vi "TCH Golbal.vi"() -> ()   [LabVIEW 2017]
panel:
  in  "秒进位":dbl
  in  "SweepCounter":i32
  in  "MouseFlag":bool
  in  "GetDataQE":bool
  in  "CloseSetVI":bool
  out "图像数据":i32[][](array[numeric])
  in  "read time":dbl
  in  "是否获取图片":dbl
  in  "Getimage flg":bool
  in  "曝光时间":dbl
  in  "Resolution flg":bool
  in  "位置保存次数":i32
  in  "结果保存次数":i32
  in  "累积位置":cluster{"X":i32, "Y":i32, "Z":i32}
  in  "ZeroFlag":cluster{"X":bool, "Y":bool, "Z":bool}
  in  "位置记录":cluster{"X":i32, "Y":i32, "Z":i32}[](array[cluster])
  in  "Clear位置":cluster{"X":i32, "Y":i32, "Z":i32}
  in  "原点":cluster{"X":i32, "Y":i32, "z":i32}
  in  "ExposureFlag":bool
  in  "Manual Color Palette":cluster{"Red":u8, "Green":u8, "Blue":u8}[](array[cluster])=[{"Red"=0, "Green"=0, "Blue"=0}, {"Red"=0, "Green"=0, "Blue"=0}, {"Red"=0, "Green"=0, "Blue"=0}, {"Red"=0, "Green"=0, "Blue"=0}, {"Red"=0, "Green"=0, "Blue"=0}, {"Red"=0, "Green"=0, "Blue"=0}, {"Red"=0, "Green"=0, "Blue"=0}, {"Red"=0, "Green"=0, "Blue"=0}, {"Red"=0, "Green"=0, "Blue"=0}, {"Red"=0, "Green"=0, "Blue"=0}, {"Red"=0, "Green"=0, "Blue"=0}, {"Red"=0, "Green"=0, "Blue"=0}, {"Red"=0, "Green"=0, "Blue"=0}, {"Red"=0, "Green"=0, "Blue"=0}, {"Red"=0, "Green"=0, "Blue"=0}, {"Red"=0, "Green"=0, "Blue"=0}, {"Red"=0, "Green"=0, "Blue"=0}, {"Red"=0, "Green"=0, "Blue"=0}, {"Red"=0, "Green"=0, "Blue"=0}, {"Red"=0, "Green"=0, "Blue"=0}, {"Red"=0, "Green"=0, "Blue"=0}, {"Red"=0, "Green"=0, "Blue"=0}, {"Red"=0, "Green"=0, "Blue"=0}, {"Red"=0, "Green"=0, "Blue"=0}, {"Red"=0, "Green"=0, "Blue"=0}, {"Red"=0, "Green"=0, "Blue"=0}, {"Red"=0, "Green"=0, "Blue"=0}, {"Red"=0, "Green"=0, "Blue"=0}, {"Red"=0, "Green"=0, "Blue"=0}, {"Red"=0, "Green"=0, "Blue"=0}, {"Red"=0, "Green"=0, "Blue"=0}, {"Red"=0, "Green"=0, "Blue"=0}, {"Red"=0, "Green"=0, "Blue"=0}, {"Red"=0, "Green"=0, "Blue"=0}, {"Red"=0, "Green"=0, "Blue"=0}, {"Red"=0, "Green"=0, "Blue"=0}, {"Red"=0, "Green"=0, "Blue"=0}, {"Red"=0, "Green"=0, "Blue"=0}, {"Red"=0, "Green"=0, "Blue"=0}, {"Red"=0, "Green"=0, "Blue"=0}, {"Red"=0, "Green"=0, "Blue"=0}, {"Red"=0, "Green"=0, "Blue"=0}, {"Red"=0, "Green"=0, "Blue"=0}, {"Red"=0, "Green"=0, "Blue"=0}, {"Red"=0, "Green"=0, "Blue"=0}, {"Red"=0, "Green"=0, "Blue"=0}, {"Red"=0, "Green"=0, "Blue"=0}, {"Red"=0, "Green"=0, "Blue"=0}, {"Red"=0, "Green"=0, "Blue"=0}, {"Red"=0, "Green"=0, "Blue"=0}, {"Red"=0, "Green"=0, "Blue"=0}, {"Red"=0, "Green"=0, "Blue"=0}, {"Red"=0, "Green"=0, "Blue"=0}, {"Red"=0, "Green"=0, "Blue"=0}, {"Red"=0, "Green"=0, "Blue"=0}, {"Red"=0, "Green"=0, "Blue"=0}, {"Red"=0, "Green"=0, "Blue"=0}, {"Red"=0, "Green"=0, "Blue"=0}, {"Red"=0, "Green"=0, "Blue"=0}, {"Red"=0, "Green"=0, "Blue"=0}, {"Red"=0, "Green"=0, "Blue"=0}, {"Red"=0, "Green"=0, "Blue"=0}, {"Red"=0, "Green"=0, "Blue"=0}, {"Red"=0, "Green"=0, "Blue"=0}, {"Red"=0, "Green"=0, "Blue"=0}, {"Red"=0, "Green"=0, "Blue"=0}, {"Red"=0, "Green"=0, "Blue"=0}, {"Red"=0, "Green"=0, "Blue"=0}, {"Red"=0, "Green"=0, "Blue"=0}, {"Red"=0, "Green"=0, "Blue"=0}, {"Red"=0, "Green"=0, "Blue"=0}, {"Red"=0, "Green"=0, "Blue"=0}, {"Red"=0, "Green"=0, "Blue"=0}, {"Red"=0, "Green"=0, "Blue"=0}, {"Red"=0, "Green"=0, "Blue"=0}, {"Red"=0, "Green"=0, "Blue"=0}, {"Red"=0, "Green"=0, "Blue"=0}, {"Red"=0, "Green"=0, "Blue"=0}, {"Red"=0, "Green"=0, "Blue"=0}, {"Red"=0, "Green"=0, "Blue"=0}, {"Red"=0, "Green"=0, "Blue"=0}, {"Red"=0, "Green"=0, "Blue"=0}, {"Red"=0, "Green"=0, "Blue"=0}, {"Red"=0, "Green"=0, "Blue"=0}, {"Red"=0, "Green"=0, "Blue"=0}, {"Red"=0, "Green"=0, "Blue"=0}, {"Red"=0, "Green"=0, "Blue"=0}, {"Red"=0, "Green"=0, "Blue"=0}, {"Red"=0, "Green"=0, "Blue"=0}, {"Red"=0, "Green"=0, "Blue"=0}, {"Red"=0, "Green"=0, "Blue"=0}, {"Red"=0, "Green"=0, "Blue"=0}, {"Red"=0, "Green"=0, "Blue"=0}, {"Red"=0, "Green"=0, "Blue"=0}, {"Red"=0, "Green"=0, "Blue"=0}, {"Red"=0, "Green"=0, "Blue"=0}, {"Red"=0, "Green"=0, "Blue"=0}, {"Red"=0, "Green"=0, "Blue"=0}, {"Red"=0, "Green"=0, "Blue"=0}, {"Red"=0, "Green"=0, "Blue"=0}, {"Red"=0, "Green"=0, "Blue"=0}, {"Red"=0, "Green"=0, "Blue"=0}, {"Red"=0, "Green"=0, "Blue"=0}, {"Red"=0, "Green"=0, "Blue"=0}, {"Red"=0, "Green"=0, "Blue"=0}, {"Red"=0, "Green"=0, "Blue"=0}, {"Red"=0, "Green"=0, "Blue"=0}, {"Red"=0, "Green"=0, "Blue"=0}, {"Red"=0, "Green"=0, "Blue"=0}, {"Red"=0, "Green"=0, "Blue"=0}, {"Red"=0, "Green"=0, "Blue"=0}, {"Red"=0, "Green"=0, "Blue"=0}, {"Red"=0, "Green"=0, "Blue"=0}, {"Red"=0, "Green"=0, "Blue"=0}, {"Red"=0, "Green"=0, "Blue"=0}, {"Red"=0, "Green"=0, "Blue"=0}, {"Red"=0, "Green"=0, "Blue"=0}, {"Red"=0, "Green"=0, "Blue"=0}, {"Red"=0, "Green"=0, "Blue"=0}, {"Red"=0, "Green"=0, "Blue"=0}, {"Red"=0, "Green"=0, "Blue"=0}, {"Red"=0, "Green"=0, "Blue"=0}, {"Red"=0, "Green"=0, "Blue"=0}, {"Red"=0, "Green"=0, "Blue"=0}, {"Red"=0, "Green"=0, "Blue"=0}, {"Red"=0, "Green"=0, "Blue"=0}, {"Red"=0, "Green"=0, "Blue"=0}, {"Red"=0, "Green"=0, "Blue"=0}, {"Red"=0, "Green"=255, "Blue"=0}, {"Red"=4, "Green"=255, "Blue"=0}, {"Red"=8, "Green"=255, "Blue"=0}, {"Red"=12, "Green"=255, "Blue"=0}, {"Red"=16, "Green"=255, "Blue"=0}, {"Red"=20, "Green"=255, "Blue"=0}, {"Red"=24, "Green"=255, "Blue"=0}, {"Red"=28, "Green"=255, "Blue"=0}, {"Red"=32, "Green"=255, "Blue"=0}, {"Red"=36, "Green"=255, "Blue"=0}, {"Red"=40, "Green"=255, "Blue"=0}, {"Red"=44, "Green"=255, "Blue"=0}, {"Red"=48, "Green"=255, "Blue"=0}, {"Red"=52, "Green"=255, "Blue"=0}, {"Red"=56, "Green"=255, "Blue"=0}, {"Red"=60, "Green"=255, "Blue"=0}, {"Red"=64, "Green"=255, "Blue"=0}, {"Red"=68, "Green"=255, "Blue"=0}, {"Red"=72, "Green"=255, "Blue"=0}, {"Red"=76, "Green"=255, "Blue"=0}, {"Red"=80, "Green"=255, "Blue"=0}, {"Red"=84, "Green"=255, "Blue"=0}, {"Red"=88, "Green"=255, "Blue"=0}, {"Red"=92, "Green"=255, "Blue"=0}, {"Red"=96, "Green"=255, "Blue"=0}, {"Red"=100, "Green"=255, "Blue"=0}, {"Red"=104, "Green"=255, "Blue"=0}, {"Red"=108, "Green"=255, "Blue"=0}, {"Red"=112, "Green"=255, "Blue"=0}, {"Red"=116, "Green"=255, "Blue"=0}, {"Red"=120, "Green"=255, "Blue"=0}, {"Red"=124, "Green"=255, "Blue"=0}, {"Red"=128, "Green"=255, "Blue"=0}, {"Red"=132, "Green"=255, "Blue"=0}, {"Red"=136, "Green"=255, "Blue"=0}, {"Red"=140, "Green"=255, "Blue"=0}, {"Red"=144, "Green"=255, "Blue"=0}, {"Red"=148, "Green"=255, "Blue"=0}, {"Red"=152, "Green"=255, "Blue"=0}, {"Red"=156, "Green"=255, "Blue"=0}, {"Red"=160, "Green"=255, "Blue"=0}, {"Red"=164, "Green"=255, "Blue"=0}, {"Red"=168, "Green"=255, "Blue"=0}, {"Red"=172, "Green"=255, "Blue"=0}, {"Red"=176, "Green"=255, "Blue"=0}, {"Red"=180, "Green"=255, "Blue"=0}, {"Red"=184, "Green"=255, "Blue"=0}, {"Red"=188, "Green"=255, "Blue"=0}, {"Red"=192, "Green"=255, "Blue"=0}, {"Red"=196, "Green"=255, "Blue"=0}, {"Red"=200, "Green"=255, "Blue"=0}, {"Red"=204, "Green"=255, "Blue"=0}, {"Red"=208, "Green"=255, "Blue"=0}, {"Red"=212, "Green"=255, "Blue"=0}, {"Red"=216, "Green"=255, "Blue"=0}, {"Red"=220, "Green"=255, "Blue"=0}, {"Red"=224, "Green"=255, "Blue"=0}, {"Red"=228, "Green"=255, "Blue"=0}, {"Red"=232, "Green"=255, "Blue"=0}, {"Red"=236, "Green"=255, "Blue"=0}, {"Red"=240, "Green"=255, "Blue"=0}, {"Red"=244, "Green"=255, "Blue"=0}, {"Red"=248, "Green"=255, "Blue"=0}, {"Red"=252, "Green"=255, "Blue"=0}, {"Red"=255, "Green"=255, "Blue"=0}, {"Red"=255, "Green"=251, "Blue"=0}, {"Red"=255, "Green"=247, "Blue"=0}, {"Red"=255, "Green"=243, "Blue"=0}, {"Red"=255, "Green"=239, "Blue"=0}, {"Red"=255, "Green"=235, "Blue"=0}, {"Red"=255, "Green"=231, "Blue"=0}, {"Red"=255, "Green"=227, "Blue"=0}, {"Red"=255, "Green"=223, "Blue"=0}, {"Red"=255, "Green"=219, "Blue"=0}, {"Red"=255, "Green"=215, "Blue"=0}, {"Red"=255, "Green"=211, "Blue"=0}, {"Red"=255, "Green"=207, "Blue"=0}, {"Red"=255, "Green"=203, "Blue"=0}, {"Red"=255, "Green"=199, "Blue"=0}, {"Red"=255, "Green"=195, "Blue"=0}, {"Red"=255, "Green"=191, "Blue"=0}, {"Red"=255, "Green"=187, "Blue"=0}, {"Red"=255, "Green"=183, "Blue"=0}, {"Red"=255, "Green"=179, "Blue"=0}, {"Red"=255, "Green"=175, "Blue"=0}, {"Red"=255, "Green"=171, "Blue"=0}, {"Red"=255, "Green"=167, "Blue"=0}, {"Red"=255, "Green"=163, "Blue"=0}, {"Red"=255, "Green"=159, "Blue"=0}, {"Red"=255, "Green"=155, "Blue"=0}, {"Red"=255, "Green"=151, "Blue"=0}, {"Red"=255, "Green"=147, "Blue"=0}, {"Red"=255, "Green"=143, "Blue"=0}, {"Red"=255, "Green"=139, "Blue"=0}, {"Red"=255, "Green"=135, "Blue"=0}, {"Red"=255, "Green"=131, "Blue"=0}, {"Red"=255, "Green"=127, "Blue"=0}, {"Red"=255, "Green"=123, "Blue"=0}, {"Red"=255, "Green"=119, "Blue"=0}, {"Red"=255, "Green"=115, "Blue"=0}, {"Red"=255, "Green"=111, "Blue"=0}, {"Red"=255, "Green"=107, "Blue"=0}, {"Red"=255, "Green"=103, "Blue"=0}, {"Red"=255, "Green"=99, "Blue"=0}, {"Red"=255, "Green"=95, "Blue"=0}, {"Red"=255, "Green"=91, "Blue"=0}, {"Red"=255, "Green"=87, "Blue"=0}, {"Red"=255, "Green"=83, "Blue"=0}, {"Red"=255, "Green"=79, "Blue"=0}, {"Red"=255, "Green"=75, "Blue"=0}, {"Red"=255, "Green"=71, "Blue"=0}, {"Red"=255, "Green"=67, "Blue"=0}, {"Red"=255, "Green"=63, "Blue"=0}, {"Red"=255, "Green"=59, "Blue"=0}, {"Red"=255, "Green"=55, "Blue"=0}, {"Red"=255, "Green"=51, "Blue"=0}, {"Red"=255, "Green"=47, "Blue"=0}, {"Red"=255, "Green"=43, "Blue"=0}, {"Red"=255, "Green"=39, "Blue"=0}, {"Red"=255, "Green"=35, "Blue"=0}, {"Red"=255, "Green"=31, "Blue"=0}, {"Red"=255, "Green"=27, "Blue"=0}, {"Red"=255, "Green"=23, "Blue"=0}, {"Red"=255, "Green"=19, "Blue"=0}, {"Red"=255, "Green"=15, "Blue"=0}, {"Red"=255, "Green"=11, "Blue"=0}, {"Red"=255, "Green"=7, "Blue"=0}, {"Red"=255, "Green"=3, "Blue"=0}]
  in  "Auto Color Palette":cluster{"Red":u8, "Green":u8, "Blue":u8}[](array[cluster])=[{"Red"=0, "Green"=0, "Blue"=0}, {"Red"=0, "Green"=0, "Blue"=0}, {"Red"=0, "Green"=0, "Blue"=0}, {"Red"=0, "Green"=0, "Blue"=0}, {"Red"=0, "Green"=0, "Blue"=0}, {"Red"=0, "Green"=0, "Blue"=0}, {"Red"=0, "Green"=0, "Blue"=0}, {"Red"=0, "Green"=0, "Blue"=0}, {"Red"=0, "Green"=0, "Blue"=0}, {"Red"=0, "Green"=0, "Blue"=0}, {"Red"=0, "Green"=0, "Blue"=0}, {"Red"=0, "Green"=0, "Blue"=0}, {"Red"=0, "Green"=0, "Blue"=0}, {"Red"=0, "Green"=0, "Blue"=0}, {"Red"=0, "Green"=0, "Blue"=0}, {"Red"=0, "Green"=0, "Blue"=0}, {"Red"=0, "Green"=0, "Blue"=0}, {"Red"=0, "Green"=0, "Blue"=0}, {"Red"=0, "Green"=0, "Blue"=0}, {"Red"=0, "Green"=0, "Blue"=0}, {"Red"=0, "Green"=0, "Blue"=0}, {"Red"=0, "Green"=0, "Blue"=0}, {"Red"=0, "Green"=0, "Blue"=0}, {"Red"=0, "Green"=0, "Blue"=0}, {"Red"=0, "Green"=0, "Blue"=0}, {"Red"=0, "Green"=0, "Blue"=0}, {"Red"=0, "Green"=0, "Blue"=0}, {"Red"=0, "Green"=0, "Blue"=0}, {"Red"=0, "Green"=0, "Blue"=0}, {"Red"=0, "Green"=0, "Blue"=0}, {"Red"=0, "Green"=0, "Blue"=0}, {"Red"=0, "Green"=0, "Blue"=0}, {"Red"=0, "Green"=0, "Blue"=0}, {"Red"=0, "Green"=0, "Blue"=0}, {"Red"=0, "Green"=0, "Blue"=0}, {"Red"=0, "Green"=0, "Blue"=0}, {"Red"=0, "Green"=0, "Blue"=0}, {"Red"=0, "Green"=0, "Blue"=0}, {"Red"=0, "Green"=0, "Blue"=0}, {"Red"=0, "Green"=0, "Blue"=0}, {"Red"=0, "Green"=0, "Blue"=0}, {"Red"=0, "Green"=0, "Blue"=0}, {"Red"=0, "Green"=0, "Blue"=0}, {"Red"=0, "Green"=0, "Blue"=0}, {"Red"=0, "Green"=0, "Blue"=0}, {"Red"=0, "Green"=0, "Blue"=0}, {"Red"=0, "Green"=0, "Blue"=0}, {"Red"=0, "Green"=0, "Blue"=0}, {"Red"=0, "Green"=0, "Blue"=0}, {"Red"=0, "Green"=0, "Blue"=0}, {"Red"=0, "Green"=0, "Blue"=0}, {"Red"=0, "Green"=0, "Blue"=0}, {"Red"=0, "Green"=0, "Blue"=0}, {"Red"=0, "Green"=0, "Blue"=0}, {"Red"=0, "Green"=0, "Blue"=0}, {"Red"=0, "Green"=0, "Blue"=0}, {"Red"=0, "Green"=0, "Blue"=0}, {"Red"=0, "Green"=0, "Blue"=0}, {"Red"=0, "Green"=0, "Blue"=0}, {"Red"=0, "Green"=0, "Blue"=0}, {"Red"=0, "Green"=0, "Blue"=0}, {"Red"=0, "Green"=0, "Blue"=0}, {"Red"=0, "Green"=0, "Blue"=0}, {"Red"=0, "Green"=0, "Blue"=0}, {"Red"=0, "Green"=0, "Blue"=0}, {"Red"=0, "Green"=0, "Blue"=0}, {"Red"=0, "Green"=0, "Blue"=0}, {"Red"=0, "Green"=0, "Blue"=0}, {"Red"=0, "Green"=0, "Blue"=0}, {"Red"=0, "Green"=0, "Blue"=0}, {"Red"=0, "Green"=0, "Blue"=0}, {"Red"=0, "Green"=0, "Blue"=0}, {"Red"=0, "Green"=0, "Blue"=0}, {"Red"=0, "Green"=0, "Blue"=0}, {"Red"=0, "Green"=0, "Blue"=0}, {"Red"=0, "Green"=0, "Blue"=0}, {"Red"=0, "Green"=0, "Blue"=0}, {"Red"=0, "Green"=0, "Blue"=0}, {"Red"=0, "Green"=0, "Blue"=0}, {"Red"=0, "Green"=0, "Blue"=0}, {"Red"=0, "Green"=0, "Blue"=0}, {"Red"=0, "Green"=0, "Blue"=0}, {"Red"=0, "Green"=0, "Blue"=0}, {"Red"=0, "Green"=0, "Blue"=0}, {"Red"=0, "Green"=0, "Blue"=0}, {"Red"=0, "Green"=0, "Blue"=0}, {"Red"=0, "Green"=0, "Blue"=0}, {"Red"=0, "Green"=0, "Blue"=0}, {"Red"=0, "Green"=0, "Blue"=0}, {"Red"=0, "Green"=0, "Blue"=0}, {"Red"=0, "Green"=0, "Blue"=0}, {"Red"=0, "Green"=0, "Blue"=0}, {"Red"=0, "Green"=0, "Blue"=0}, {"Red"=0, "Green"=0, "Blue"=0}, {"Red"=0, "Green"=0, "Blue"=0}, {"Red"=0, "Green"=0, "Blue"=0}, {"Red"=0, "Green"=0, "Blue"=0}, {"Red"=0, "Green"=0, "Blue"=0}, {"Red"=0, "Green"=0, "Blue"=0}, {"Red"=0, "Green"=0, "Blue"=0}, {"Red"=0, "Green"=0, "Blue"=0}, {"Red"=0, "Green"=0, "Blue"=0}, {"Red"=0, "Green"=0, "Blue"=0}, {"Red"=0, "Green"=0, "Blue"=0}, {"Red"=0, "Green"=0, "Blue"=0}, {"Red"=0, "Green"=0, "Blue"=0}, {"Red"=0, "Green"=0, "Blue"=0}, {"Red"=0, "Green"=0, "Blue"=0}, {"Red"=0, "Green"=0, "Blue"=0}, {"Red"=0, "Green"=0, "Blue"=0}, {"Red"=0, "Green"=0, "Blue"=0}, {"Red"=0, "Green"=0, "Blue"=0}, {"Red"=0, "Green"=0, "Blue"=0}, {"Red"=0, "Green"=0, "Blue"=0}, {"Red"=0, "Green"=0, "Blue"=0}, {"Red"=0, "Green"=0, "Blue"=0}, {"Red"=0, "Green"=0, "Blue"=0}, {"Red"=0, "Green"=0, "Blue"=0}, {"Red"=0, "Green"=0, "Blue"=0}, {"Red"=0, "Green"=0, "Blue"=0}, {"Red"=0, "Green"=0, "Blue"=0}, {"Red"=0, "Green"=0, "Blue"=0}, {"Red"=0, "Green"=0, "Blue"=0}, {"Red"=0, "Green"=0, "Blue"=0}, {"Red"=0, "Green"=0, "Blue"=0}, {"Red"=0, "Green"=0, "Blue"=0}, {"Red"=0, "Green"=0, "Blue"=0}, {"Red"=0, "Green"=0, "Blue"=0}, {"Red"=0, "Green"=255, "Blue"=0}, {"Red"=4, "Green"=255, "Blue"=0}, {"Red"=8, "Green"=255, "Blue"=0}, {"Red"=12, "Green"=255, "Blue"=0}, {"Red"=16, "Green"=255, "Blue"=0}, {"Red"=20, "Green"=255, "Blue"=0}, {"Red"=24, "Green"=255, "Blue"=0}, {"Red"=28, "Green"=255, "Blue"=0}, {"Red"=32, "Green"=255, "Blue"=0}, {"Red"=36, "Green"=255, "Blue"=0}, {"Red"=40, "Green"=255, "Blue"=0}, {"Red"=44, "Green"=255, "Blue"=0}, {"Red"=48, "Green"=255, "Blue"=0}, {"Red"=52, "Green"=255, "Blue"=0}, {"Red"=56, "Green"=255, "Blue"=0}, {"Red"=60, "Green"=255, "Blue"=0}, {"Red"=64, "Green"=255, "Blue"=0}, {"Red"=68, "Green"=255, "Blue"=0}, {"Red"=72, "Green"=255, "Blue"=0}, {"Red"=76, "Green"=255, "Blue"=0}, {"Red"=80, "Green"=255, "Blue"=0}, {"Red"=84, "Green"=255, "Blue"=0}, {"Red"=88, "Green"=255, "Blue"=0}, {"Red"=92, "Green"=255, "Blue"=0}, {"Red"=96, "Green"=255, "Blue"=0}, {"Red"=100, "Green"=255, "Blue"=0}, {"Red"=104, "Green"=255, "Blue"=0}, {"Red"=108, "Green"=255, "Blue"=0}, {"Red"=112, "Green"=255, "Blue"=0}, {"Red"=116, "Green"=255, "Blue"=0}, {"Red"=120, "Green"=255, "Blue"=0}, {"Red"=124, "Green"=255, "Blue"=0}, {"Red"=128, "Green"=255, "Blue"=0}, {"Red"=132, "Green"=255, "Blue"=0}, {"Red"=136, "Green"=255, "Blue"=0}, {"Red"=140, "Green"=255, "Blue"=0}, {"Red"=144, "Green"=255, "Blue"=0}, {"Red"=148, "Green"=255, "Blue"=0}, {"Red"=152, "Green"=255, "Blue"=0}, {"Red"=156, "Green"=255, "Blue"=0}, {"Red"=160, "Green"=255, "Blue"=0}, {"Red"=164, "Green"=255, "Blue"=0}, {"Red"=168, "Green"=255, "Blue"=0}, {"Red"=172, "Green"=255, "Blue"=0}, {"Red"=176, "Green"=255, "Blue"=0}, {"Red"=180, "Green"=255, "Blue"=0}, {"Red"=184, "Green"=255, "Blue"=0}, {"Red"=188, "Green"=255, "Blue"=0}, {"Red"=192, "Green"=255, "Blue"=0}, {"Red"=196, "Green"=255, "Blue"=0}, {"Red"=200, "Green"=255, "Blue"=0}, {"Red"=204, "Green"=255, "Blue"=0}, {"Red"=208, "Green"=255, "Blue"=0}, {"Red"=212, "Green"=255, "Blue"=0}, {"Red"=216, "Green"=255, "Blue"=0}, {"Red"=220, "Green"=255, "Blue"=0}, {"Red"=224, "Green"=255, "Blue"=0}, {"Red"=228, "Green"=255, "Blue"=0}, {"Red"=232, "Green"=255, "Blue"=0}, {"Red"=236, "Green"=255, "Blue"=0}, {"Red"=240, "Green"=255, "Blue"=0}, {"Red"=244, "Green"=255, "Blue"=0}, {"Red"=248, "Green"=255, "Blue"=0}, {"Red"=252, "Green"=255, "Blue"=0}, {"Red"=255, "Green"=255, "Blue"=0}, {"Red"=255, "Green"=251, "Blue"=0}, {"Red"=255, "Green"=247, "Blue"=0}, {"Red"=255, "Green"=243, "Blue"=0}, {"Red"=255, "Green"=239, "Blue"=0}, {"Red"=255, "Green"=235, "Blue"=0}, {"Red"=255, "Green"=231, "Blue"=0}, {"Red"=255, "Green"=227, "Blue"=0}, {"Red"=255, "Green"=223, "Blue"=0}, {"Red"=255, "Green"=219, "Blue"=0}, {"Red"=255, "Green"=215, "Blue"=0}, {"Red"=255, "Green"=211, "Blue"=0}, {"Red"=255, "Green"=207, "Blue"=0}, {"Red"=255, "Green"=203, "Blue"=0}, {"Red"=255, "Green"=199, "Blue"=0}, {"Red"=255, "Green"=195, "Blue"=0}, {"Red"=255, "Green"=191, "Blue"=0}, {"Red"=255, "Green"=187, "Blue"=0}, {"Red"=255, "Green"=183, "Blue"=0}, {"Red"=255, "Green"=179, "Blue"=0}, {"Red"=255, "Green"=175, "Blue"=0}, {"Red"=255, "Green"=171, "Blue"=0}, {"Red"=255, "Green"=167, "Blue"=0}, {"Red"=255, "Green"=163, "Blue"=0}, {"Red"=255, "Green"=159, "Blue"=0}, {"Red"=255, "Green"=155, "Blue"=0}, {"Red"=255, "Green"=151, "Blue"=0}, {"Red"=255, "Green"=147, "Blue"=0}, {"Red"=255, "Green"=143, "Blue"=0}, {"Red"=255, "Green"=139, "Blue"=0}, {"Red"=255, "Green"=135, "Blue"=0}, {"Red"=255, "Green"=131, "Blue"=0}, {"Red"=255, "Green"=127, "Blue"=0}, {"Red"=255, "Green"=123, "Blue"=0}, {"Red"=255, "Green"=119, "Blue"=0}, {"Red"=255, "Green"=115, "Blue"=0}, {"Red"=255, "Green"=111, "Blue"=0}, {"Red"=255, "Green"=107, "Blue"=0}, {"Red"=255, "Green"=103, "Blue"=0}, {"Red"=255, "Green"=99, "Blue"=0}, {"Red"=255, "Green"=95, "Blue"=0}, {"Red"=255, "Green"=91, "Blue"=0}, {"Red"=255, "Green"=87, "Blue"=0}, {"Red"=255, "Green"=83, "Blue"=0}, {"Red"=255, "Green"=79, "Blue"=0}, {"Red"=255, "Green"=75, "Blue"=0}, {"Red"=255, "Green"=71, "Blue"=0}, {"Red"=255, "Green"=67, "Blue"=0}, {"Red"=255, "Green"=63, "Blue"=0}, {"Red"=255, "Green"=59, "Blue"=0}, {"Red"=255, "Green"=55, "Blue"=0}, {"Red"=255, "Green"=51, "Blue"=0}, {"Red"=255, "Green"=47, "Blue"=0}, {"Red"=255, "Green"=43, "Blue"=0}, {"Red"=255, "Green"=39, "Blue"=0}, {"Red"=255, "Green"=35, "Blue"=0}, {"Red"=255, "Green"=31, "Blue"=0}, {"Red"=255, "Green"=27, "Blue"=0}, {"Red"=255, "Green"=23, "Blue"=0}, {"Red"=255, "Green"=19, "Blue"=0}, {"Red"=255, "Green"=15, "Blue"=0}, {"Red"=255, "Green"=11, "Blue"=0}, {"Red"=255, "Green"=7, "Blue"=0}, {"Red"=255, "Green"=3, "Blue"=0}]
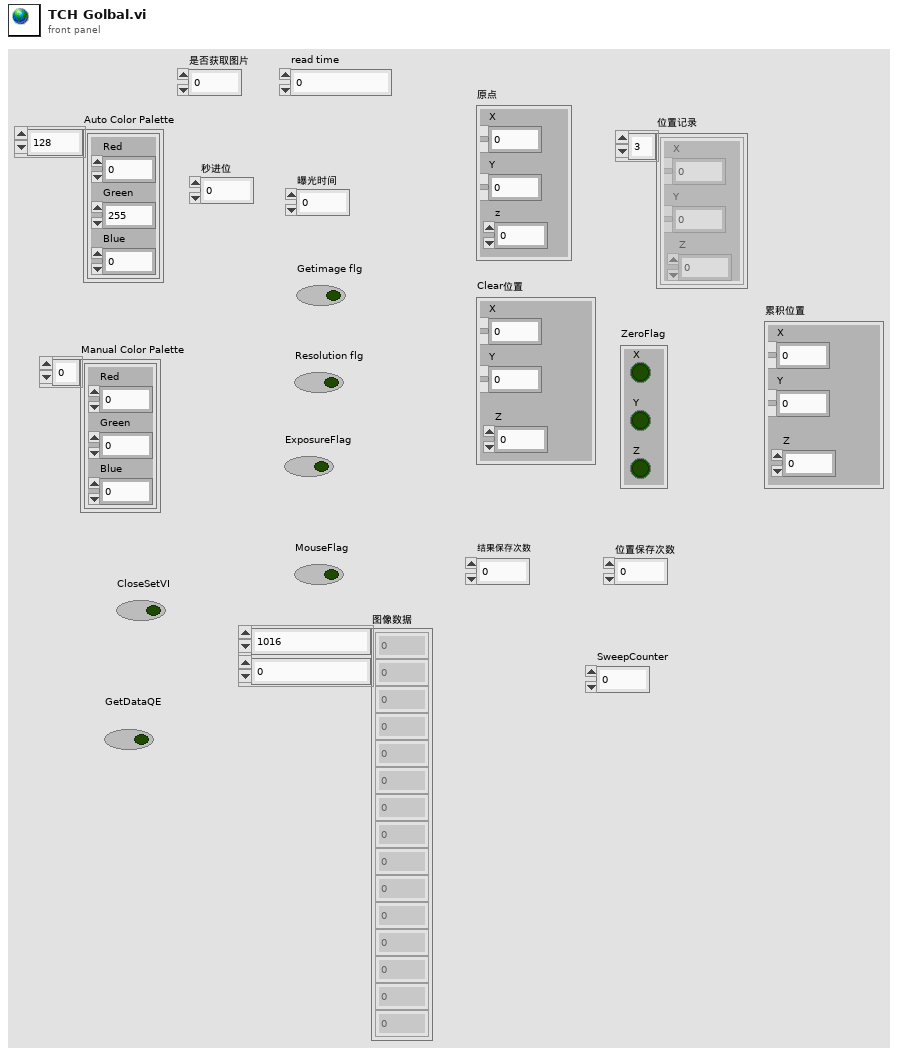
[diagram p1: front panel]
diagram:
